vi "Actuate.vi"(8 "error in":errorcluster) -> (0 "error out":errorcluster, 1 "Actuators":T1, 4 "Actuators":u32)   [LabVIEW 2017]
uses:
  Type Defs/Actuators.ctl
  <vilib>/myRIO/Instrument Drivers/Onboard IO/DIO/typedefs/DIO Reference.ctl
  <vilib>/myRIO/Common/Instrument Driver Framework/Utilities/typedefs/myRIO Generic Hardware Reference.ctl
  <vilib>/myRIO/Common/Instrument Driver Framework/Utilities/typedefs/Hardware Version Enum.ctl
  <vilib>/myRIO/Common/Instrument Driver Framework/Utilities/typedefs/myRIO v1.0 Reference.ctl
  <vilib>/myRIO/Common/Instrument Driver Framework/Utilities/typedefs/Generic FPGA Reference.ctl
  <vilib>/myRIO/Common/Instrument Driver Framework/myRIO v1.0/DIO/typedefs/DIO Channels List.ctl
  <vilib>/myRIO/Common/Instrument Driver Framework/myRIO v1.0/DIO/typedefs/DIO Channels Enum.ctl
  <vilib>/userdefined/High Color/nirio_resource_hc.ctl
  <vilib>/myRIO/Common/Instrument Driver Framework/Utilities/vis/Is FPGA Ref Available.vi
  <vilib>/myRIO/Common/Instrument Driver Framework/myRIO v1.0/DIO/vis/myRIO v1.1 Open DIO.vi
  <vilib>/myRIO/Instrument Drivers/Onboard IO/DIO/vis/Read.vi
  <vilib>/myRIO/Common/Instrument Driver Framework/Utilities/vis/Validate Channels.vi
  <vilib>/myRIO/Common/Instrument Driver Framework/myRIO v1.0/DIO/vis/myRIO v1.0 Reserve DIO.vi
  <vilib>/myRIO/Common/Instrument Driver Framework/myRIO v1.0/Resource Manager/vis/myRIO v1.0 Reserve Channel List.vi
  <vilib>/myRIO/Common/Instrument Driver Framework/myRIO v1.0/DIO/vis/myRIO v1.0 Build MUX Configuration DIO.vi
  <vilib>/myRIO/Common/Instrument Driver Framework/myRIO v1.0/Resource Manager/vis/myRIO v1.0 Reserve Channel.vi
  <vilib>/myRIO/Common/Instrument Driver Framework/myRIO v1.0/Resource Manager/vis/myRIO v1.0 Unreserve Channel.vi
  <vilib>/myRIO/Common/Instrument Driver Framework/myRIO v1.0/Resource Manager/vis/myRIO v1.0 Create Configuration List.vi
  <vilib>/myRIO/Common/Instrument Driver Framework/myRIO v1.0/Resource Manager/vis/myRIO v1.0 Build Mutex Name.vi
  <vilib>/Utility/VariantDataType/GetNumericInfo.vi
  <vilib>/Utility/error.llb/Error Cluster From Error Code.vi
  <vilib>/myRIO/Common/Instrument Driver Framework/myRIO v1.0/myRIO v1.1 Open.vi
  <vilib>/myRIO/Common/Instrument Driver Framework/Utilities/vis/IO Manager.vi
  <vilib>/myRIO/Common/Instrument Driver Framework/Utilities/vis/Configuration Manager.vi
  <vilib>/myRIO/Common/Instrument Driver Framework/myRIO v1.0/Resource Manager/vis/myRIO v1.0 Configure IO.vi
  <vilib>/myRIO/Common/Instrument Driver Framework/myRIO v1.0/myRIO v1.0 Close.vi
  <vilib>/myRIO/Common/Instrument Driver Framework/myRIO v1.0/DIO/vis/myRIO v1.0 Read DIO.vi
  <vilib>/myRIO/Common/Instrument Driver Framework/myRIO v1.0/DIO/vis/myRIO v1.0 Write DIO.vi
  <vilib>/myRIO/Express VI/Onboard Devices/Button/Button Express VI.xnode
  <vilib>/myRIO/Instrument Drivers/Onboard IO/DIO/vis/myRIO DIO Open.xnode
  <vilib>/myRIO/Express VI/Onboard Devices/LED/LED Express VI.xnode
  <vilib>/myRIO/Instrument Drivers/Onboard IO/DIO/DIO.lvlib
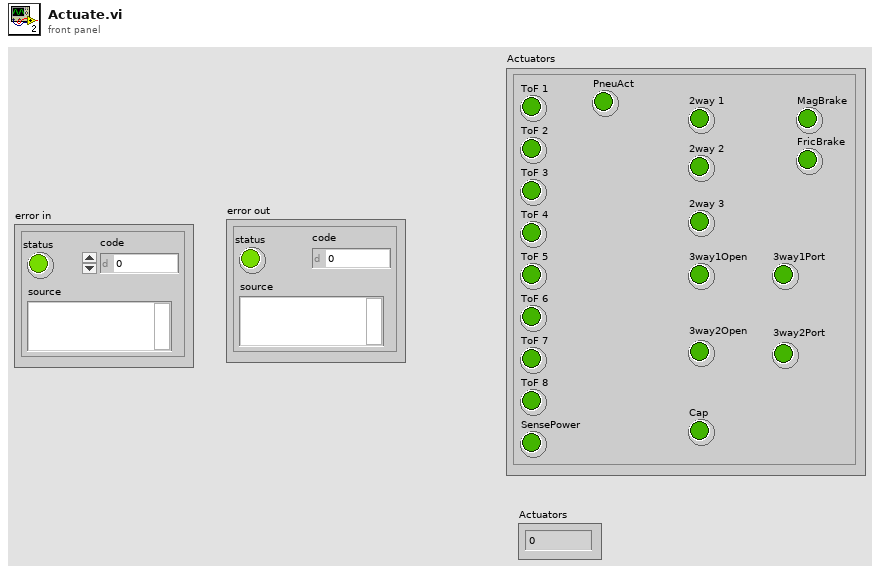
[diagram p1: front panel]
types:
  T1 = typedef "Actuators.ctl" = cluster{"2way 1":bool, "MagBrake":bool, "FricBrake":bool, "2way 2":bool, "PneuAct":bool, "2way 3":bool, "ToF 1":bool, "ToF 2":bool, "ToF 3":bool, "ToF 4":bool, "ToF 5":bool, "ToF 6":bool, "ToF 7":bool, "ToF 8":bool, "Cap":bool, "SensePower":bool, "3way1Open":bool, "3way1Port":bool, "3way2Open":bool, "3way2Port":bool}
  T2 = typedef "DIO.lvlib/DIO Reference.ctl" = cluster{"myRIO Reference":T3, "DIO Channels List":T7}
  T3 = typedef "myRIO Generic Hardware Reference.ctl" = cluster{"myRIO Model":T4, "myRIO Hardware Reference":T5}
  T4 = typedef "Hardware Version Enum.ctl" = enum16{"Unknown", "myRIO-1900", "myRIO-1950", "roboRIO", "NI ELVIS RIO CM"}
  T5 = typedef "myRIO v1.0 Reference.ctl" = cluster{"Generic FPGA Reference":T6, "Allow multiple opens":bool}
  T6 = typedef "Generic FPGA Reference.ctl" = refnum<k20>
  T7 = typedef "DIO Channels List.ctl" = T8[]
  T8 = typedef "DIO Channels Enum.ctl" = enum16{"Not Connected", "C/DIO0", "C/DIO1", "C/DIO2", "C/DIO3", "C/DIO4", "C/DIO5", "C/DIO6", "C/DIO7", "A/DIO0", "A/DIO1", "A/DIO2", "A/DIO3", "A/DIO4", "A/DIO5", "A/DIO6", "A/DIO7", "A/DIO8", "A/DIO9", "A/DIO10", "A/DIO11", "A/DIO12", "A/DIO13", "A/DIO14", "A/DIO15", "B/DIO0", "B/DIO1", "B/DIO2", "B/DIO3", "B/DIO4", "B/DIO5", "B/DIO6", "B/DIO7", "B/DIO8", "B/DIO9", "B/DIO10", "B/DIO11", "B/DIO12", "B/DIO13", "B/DIO14", "B/DIO15", "LED0", "LED1", "LED2", "LED3", "Button0", "DIO/DIO0", "DIO/DIO1", "DIO/DIO2", "DIO/DIO3", "DIO/DIO4", "DIO/DIO5", "DIO/DIO6", "DIO/DIO7", "DIO/DIO8", "DIO/DIO9", "SPI/CS0", "SPI/CS1", "SPI/CS2", "SPI/CS3", "LED RADIO (Green)", "LED RADIO (Red)", "LED COMM (Green)", "LED COMM (Red)", "LED MODE (Green)", "LED MODE (Red)"}
  T9 = cluster{"[0]":bool, "[1]":bool, "[2]":bool, "[3]":bool, "[4]":bool, "[5]":bool, "[6]":bool, "[7]":bool, "[8]":bool, "[9]":bool, "[10]":bool, "[11]":bool, "[12]":bool, "[13]":bool, "[14]":bool, "[15]":bool, "[16]":bool, "[17]":bool, "[18]":bool, "[19]":bool}
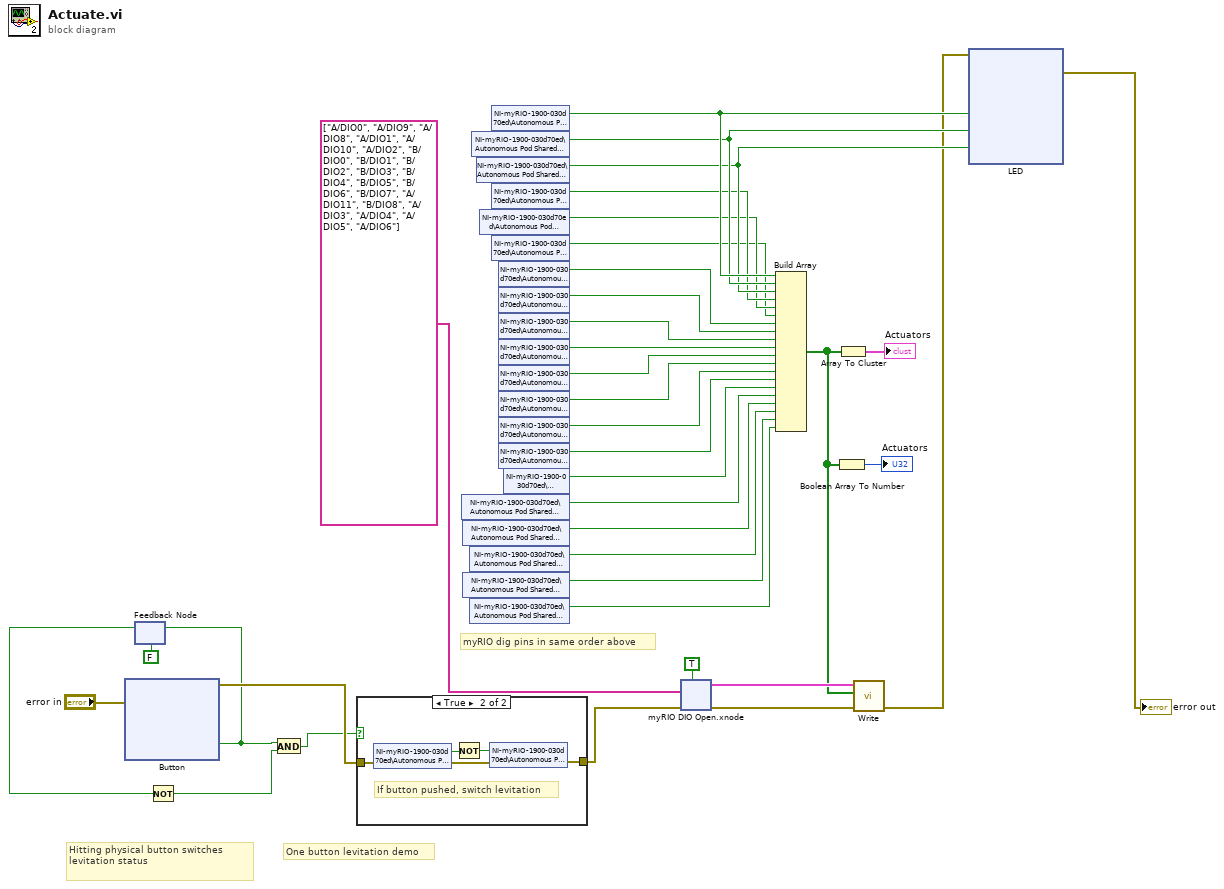
[diagram p0: block diagram]
diagram:
  # "One button levitation demo"
  # "myRIO dig pins in same order above"
  # "Hitting physical button switches levitation status"
  n1 = xnode "Button"("error in (no error)"="error in") -> ("Value"=w4:bool, "error out"=w12:errorcluster)
  n2 = feedback #1(FALSE ("Rising Edge")) -> (w2:bool)
  n3 = feedback-in #1(w4) -> ()
  n4 = Not(x=w2) -> (.not. x?=w3:bool)
  n5 = And(x=w4, y=w3) -> (x .and. y?=w1:bool)
  n6 = case shown="True" w1 {
    tunnel: w12 -> [w38 w41]
    tunnel: [w38 w39] -> w11
    frame False {
    }
    frame True {
      # "If button pushed, switch levitation"
      n7 = shared-variable "NI-myRIO-1900-030d70ed\\Autonomous Pod Shared Variables.lvlib\\2way1"(error in=w41) -> (w43:bool, error out=w40:errorcluster)
      n8 = Not(x=w43) -> (.not. x?=w42:bool)
      n9 = shared-variable "NI-myRIO-1900-030d70ed\\Autonomous Pod Shared Variables.lvlib\\2way1"(w42, error in=w40) -> (error out=w39:errorcluster)
    }
  }
  n10 = shared-variable "NI-myRIO-1900-030d70ed\\Autonomous Pod Shared Variables.lvlib\\SensePower"() -> (w32:bool)  [unwired: 1 in, 1 out]
  n11 = shared-variable "NI-myRIO-1900-030d70ed\\Autonomous Pod Shared Variables.lvlib\\3way1Open"() -> (w36:bool)  [unwired: 1 in, 1 out]
  n12 = shared-variable "NI-myRIO-1900-030d70ed\\Autonomous Pod Shared Variables.lvlib\\3way2Open"() -> (w34:bool)  [unwired: 1 in, 1 out]
  n13 = shared-variable "NI-myRIO-1900-030d70ed\\Autonomous Pod Shared Variables.lvlib\\3way1Port"() -> (w35:bool)  [unwired: 1 in, 1 out]
  n14 = shared-variable "NI-myRIO-1900-030d70ed\\Autonomous Pod Shared Variables.lvlib\\3way2Port"() -> (w33:bool)  [unwired: 1 in, 1 out]
  n15 = shared-variable "NI-myRIO-1900-030d70ed\\Autonomous Pod Shared Variables.lvlib\\MagBrake"() -> (w21:bool)  [unwired: 1 in, 1 out]
  n16 = shared-variable "NI-myRIO-1900-030d70ed\\Autonomous Pod Shared Variables.lvlib\\FricBrake"() -> (w20:bool)  [unwired: 1 in, 1 out]
  n17 = shared-variable "NI-myRIO-1900-030d70ed\\Autonomous Pod Shared Variables.lvlib\\PneuAct"() -> (w18:bool)  [unwired: 1 in, 1 out]
  n18 = shared-variable "NI-myRIO-1900-030d70ed\\Autonomous Pod Shared Variables.lvlib\\2way1"() -> (w22:bool)  [unwired: 1 in, 1 out]
  n19 = shared-variable "NI-myRIO-1900-030d70ed\\Autonomous Pod Shared Variables.lvlib\\2way2"() -> (w19:bool)  [unwired: 1 in, 1 out]
  n20 = shared-variable "NI-myRIO-1900-030d70ed\\Autonomous Pod Shared Variables.lvlib\\2way3"() -> (w17:bool)  [unwired: 1 in, 1 out]
  n21 = shared-variable "NI-myRIO-1900-030d70ed\\Autonomous Pod Shared Variables.lvlib\\ToF1"() -> (w23:bool)  [unwired: 1 in, 1 out]
  n22 = shared-variable "NI-myRIO-1900-030d70ed\\Autonomous Pod Shared Variables.lvlib\\ToF2"() -> (w24:bool)  [unwired: 1 in, 1 out]
  n23 = shared-variable "NI-myRIO-1900-030d70ed\\Autonomous Pod Shared Variables.lvlib\\ToF3"() -> (w25:bool)  [unwired: 1 in, 1 out]
  n24 = shared-variable "NI-myRIO-1900-030d70ed\\Autonomous Pod Shared Variables.lvlib\\ToF4"() -> (w26:bool)  [unwired: 1 in, 1 out]
  n25 = shared-variable "NI-myRIO-1900-030d70ed\\Autonomous Pod Shared Variables.lvlib\\ToF5"() -> (w27:bool)  [unwired: 1 in, 1 out]
  n26 = shared-variable "NI-myRIO-1900-030d70ed\\Autonomous Pod Shared Variables.lvlib\\ToF6"() -> (w28:bool)  [unwired: 1 in, 1 out]
  n27 = shared-variable "NI-myRIO-1900-030d70ed\\Autonomous Pod Shared Variables.lvlib\\ToF7"() -> (w29:bool)  [unwired: 1 in, 1 out]
  n28 = shared-variable "NI-myRIO-1900-030d70ed\\Autonomous Pod Shared Variables.lvlib\\ToF8"() -> (w30:bool)  [unwired: 1 in, 1 out]
  n29 = shared-variable "NI-myRIO-1900-030d70ed\\Autonomous Pod Shared Variables.lvlib\\Cap"() -> (w31:bool)  [unwired: 1 in, 1 out]
  n30 = xnode "myRIO DIO Open.xnode"("error in (no error)"=w11, "Allow multiple opens?"=TRUE, "Channel Names"=tag[] ["A/DIO0", "A/DIO9", "A/DIO8", "A/DIO1", "A/DIO10", "A/DIO2", "B/DIO0", "B/DIO1", "B/DIO2", "B/DIO3", "B/DIO4", "B/DIO5", "B/DIO6", "B/DIO7", "A/DIO11", "B/DIO8", "A/DIO3", "A/DIO4", "A/DIO5", "A/DIO6"]) -> ("error out"=w14:errorcluster, "DIO Ref Out"=w13:T2)
  n31 = Build Array(w22, w21, w20, w19, w18, w17, w23, w24, w25, w26, w27, w28, w29, w30, w31, w32, w36, w35, w34, w33) -> (w7:bool[])
  n32 = Boolean Array To Number(Boolean array=w7) -> (number=→"Actuators":u32)
  n33 = Array To Cluster(array=w7) -> (cluster=→"Actuators":T9)
  n34 = call <vilib>:"Write.vi"("error in (no error)"=w14, "Values"=w7, "DIO Ref In"=w13) -> ("error out"=w9:errorcluster)  [unwired: 6 in, 1 out]
  n35 = xnode "LED"("LED0"=w22, "LED1"=w21, "LED2"=w20, "error in (no error)"=w9) -> ("error out"=→"error out":errorcluster)
